vi "WPI_RobotDriveArcadeDrive.vi"   [LabVIEW 2017]
doc: "Configures the motors for arcade driving. Arcade driving uses a single joystick where the y-axis controls driving speed and the x-axis controls turning rate. This VI encodes the x-axis and y-axis values to supply different signals to each motor for turning.\n\nThis software is licensed. Open the labview\\readme\\WPI Robotics Library Open Source License.txt file for more information."
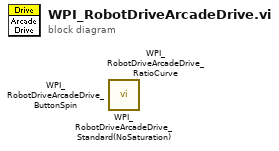
[diagram p0: block diagram]
diagram:
  n1 = call <vilib>:"WPI_RobotDriveArcadeDrive_Standard(NoSaturation).vi"() -> ()  [unwired: 9 in, 3 out]
  n2 = call <vilib>:"WPI_RobotDriveArcadeDrive_RatioCurve.vi"() -> ()  [unwired: 9 in, 3 out]
  n3 = call <vilib>:"WPI_RobotDriveArcadeDrive_ButtonSpin.vi"() -> ()  [unwired: 9 in, 3 out]
